vi "manifold config control active odor check (sub-vi).vi"(7 "active odor chanel set":set{T6}(c389), 10 "manifold config array":T1) -> (2 "manifold config error flag array":bool[][](array[boolean]))   [LabVIEW 2021]
uses:
  type-defs/odor selection (type def).ctl
  type-defs/manifold configuration cluster array (type def).ctl
  type-defs/manifold configuration cluster (type def).ctl
  type-defs/manifold selection.ctl
  type-defs/single port single odor cluster.ctl
  type-defs/port number (type def).ctl
  type-defs/odor color (type def).ctl
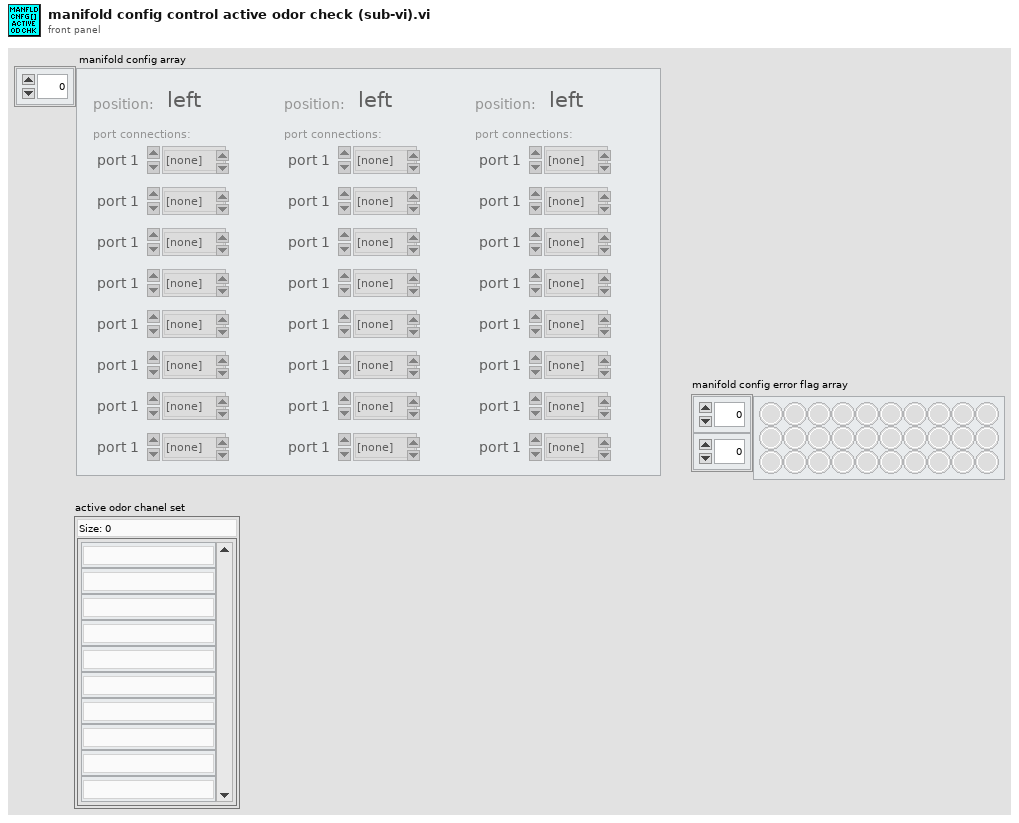
[diagram p1: front panel]
types:
  T1 = typedef "manifold configuration cluster array (type def).ctl" = T2[]
  T2 = typedef "manifold configuration cluster (type def).ctl" = cluster{"position:":T3, "port connections:":T4[]}
  T3 = typedef "manifold selection.ctl" = enum16{"left", "middle", "right"}
  T4 = typedef "single port single odor cluster.ctl" = cluster{"port number":T5, "connected odor":T6, "error":bool, "odor color":T7}
  T5 = typedef "port number (type def).ctl" = enum16{"port 1", "port 2", "port 3", "port 4", "port 5", "port 6", "port 7", "port 8"}
  T6 = typedef "odor selection (type def).ctl" = enum16{"[none]", "odor 1", "odor 2", "odor 3", "odor 4", "odor 5", "odor 6", "odor 7", "odor 8", "odor 9", "odor 10"}
  T7 = typedef "odor color (type def).ctl" = u16
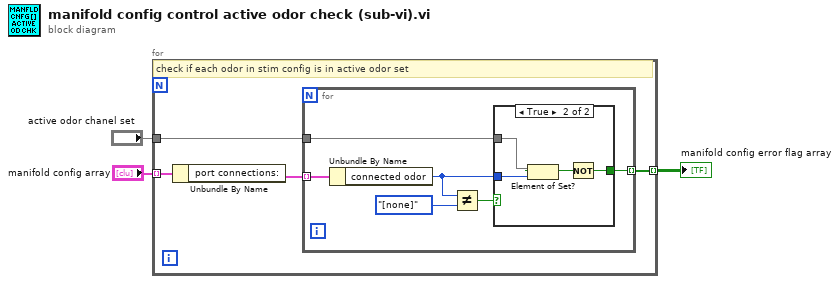
[diagram p0: block diagram]
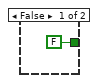
[diagram p2: hidden frame]
diagram:
  n1 = for {
    tunnel: "manifold config array" -> [w6] mode=indexing
    tunnel: "active odor chanel set" -> [w5]
    tunnel: [w4] -> w2 mode=indexing
    # "check if each odor in stim config is in active odor set"
    n2 = Unbundle By Name(w6) -> ("port connections:"=w7:T4[])
    n3 = for {
      tunnel: w7 -> [w13] mode=indexing
      tunnel: w5 -> [w9]
      tunnel: [w8] -> w4 mode=indexing
      n4 = Unbundle By Name(w13) -> ("connected odor"=w12:T6)
      n5 = Not Equal?(x=w12, y=odor_selection_(type_def)."[none]" ("connected odor")) -> (x != y?=w10:bool)
      n6 = case shown="True" w10 {
        tunnel: w12 -> [_ w17]
        tunnel: w9 -> [_ w18]
        tunnel: [FALSE w15] -> w8
        frame False {
        }
        frame True {
          n7 = Element of Set?(10:w17, 11:w18) -> (3:w16:bool)
          n8 = Not(x=w16) -> (.not. x?=w15:bool)
        }
      }
    }
  }
  "manifold config error flag array" <- w2
